vi "MQTT_TCP_Read.vi"(7 "mode (standard)":T1(ring), 8 "error in (no error)":errorcluster, 9 "timeout ms (25000)":i32=25000, 10 "bytes to read":i32=1, 11 "connection ID":refnum<k5>) -> (0 "error out":errorcluster, 2 "data out":string, 3 "connection ID out":refnum<k5>)   [LabVIEW 2012, in "MQTT_Functions.lvlib"]
uses:
  MQTT_Functions.lvlib
panel:
  # "this is just a wrapper for the TCP Read function\nadd or replace functionality as desired"
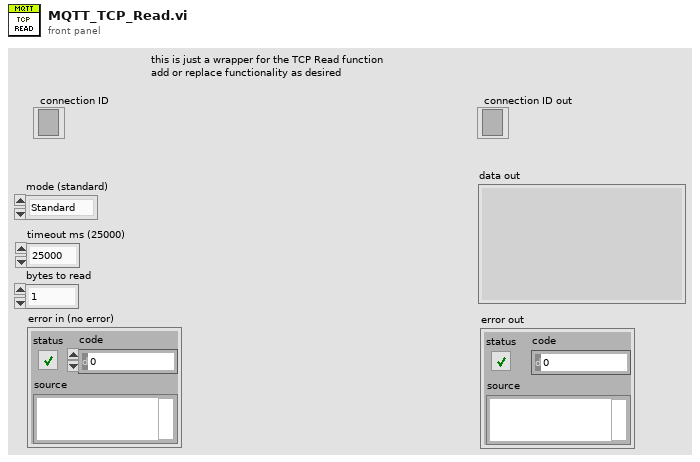
[diagram p1: front panel]
types:
  T1 = enum16{"Standard", "Buffered", "CRLF", "Immediate"}
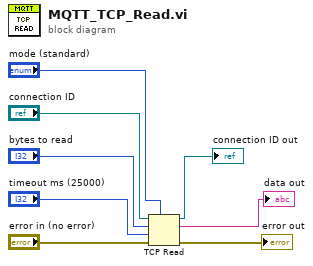
[diagram p0: block diagram]
diagram:
  n1 = TCP Read(connection ID="connection ID", bytes to read="bytes to read", error in (no error)="error in (no error)", 7:"mode (standard)", 9:"timeout ms (25000)") -> (connection ID out=→"connection ID out":refnum<k5>, data out=→"data out":string, error out=→"error out":errorcluster)
